vi "Pos ctrl window-Step increment switch.vi"(6 "Mode":enum16{"XY", "Z"}(ring), 9 "State":T1, 10 "Previous State":T1) -> (1 "Wait for acknowledge?":bool, 3 "Increment (um)":sgl)   [LabVIEW 2020]
uses:
  Typedefs/Pos Ctrl States.ctl
  Globals/Pos ctrl window globals.vi
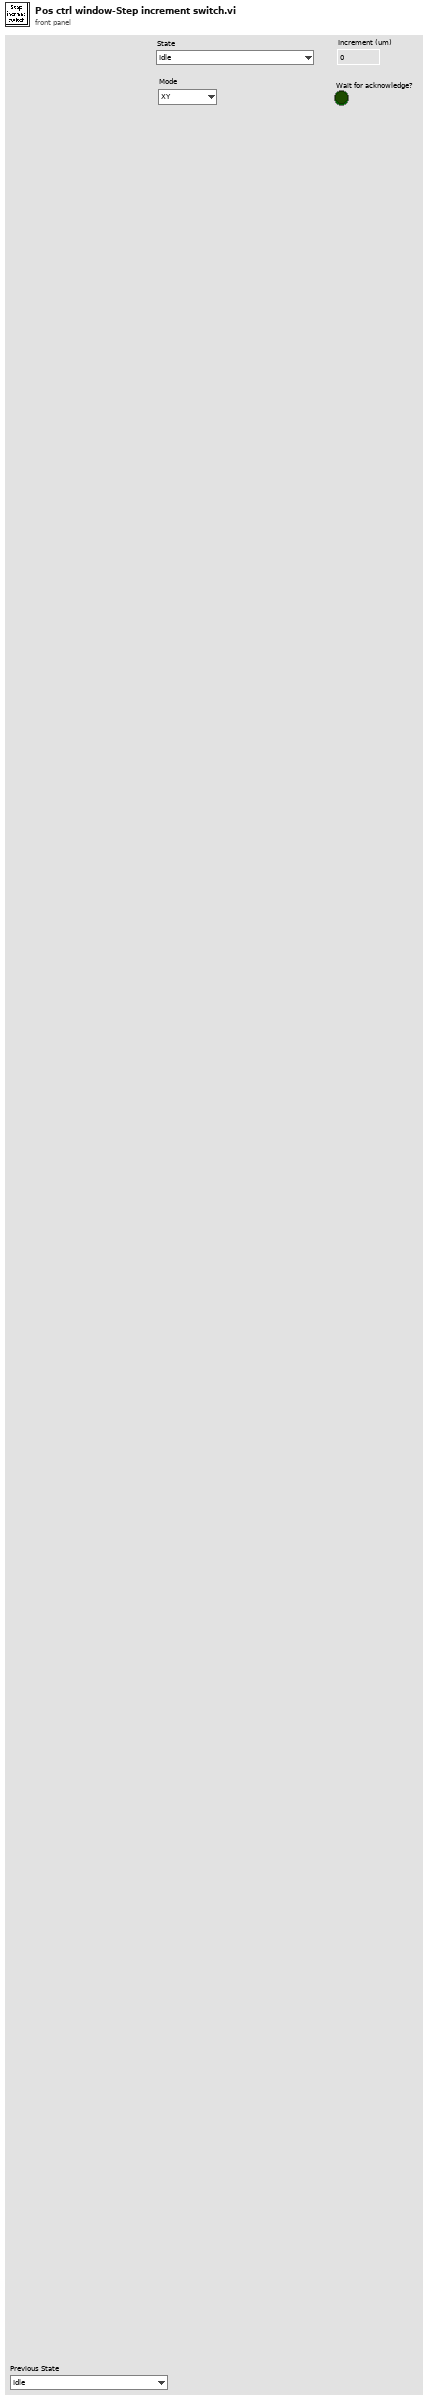
[diagram p1: front panel]
types:
  T1 = typedef "Pos Ctrl States.ctl" = enum16{"Idle", "Count-down", "Request single step (ack.)", "Request single step (no ack.)", "Request continuous movement", "Request movement stop"}
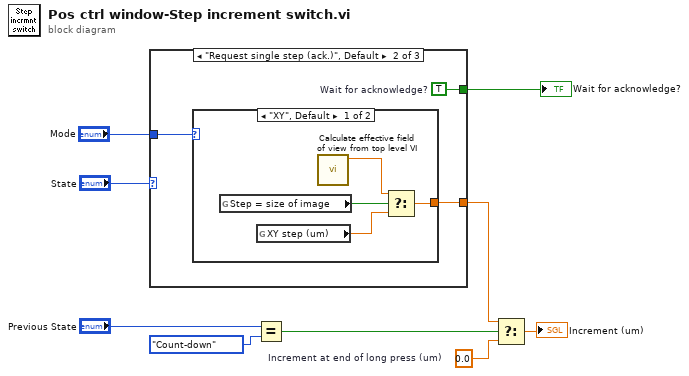
[diagram p0: block diagram]
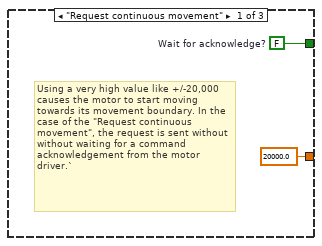
[diagram p2: hidden frame]
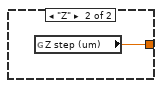
[diagram p3: hidden frame]
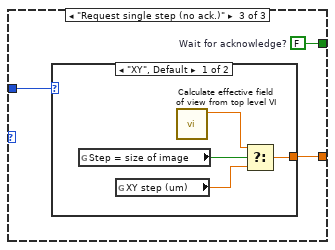
[diagram p4: hidden frame]
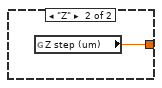
[diagram p5: hidden frame]
diagram:
  w9 = sgl 0.0  # Increment at end of long press (um)
  n1 = case shown="\"Request single step (ack.)\", Default" "State" {
    tunnel: [sgl 20000.0 ("XY step (um)") w14 w22] -> w4
    tunnel: "Mode" -> [_ w13 w21]
    tunnel: [w10 w12 w20] -> w1
    frame "Request continuous movement" {
      w10 = FALSE  # Wait for acknowledge?
      # "Using a very high value like +/-20,000 causes the motor to start moving towards its movement boundary. In the case of the \"Request continuous movement\", the request is sent without without waiting for a command acknowledgement from the motor driver.`"
    }
    frame "Request single step (ack.)", Default {
      w12 = TRUE  # Wait for acknowledge?
      n2 = case shown="\"XY\", Default" w13 {
        tunnel: [w18 w19] -> w14
        frame "XY", Default {
          n3 = global read "Pos ctrl window globals.vi" "Step = size of image"() -> (w16:bool)
          n4 = global read "Pos ctrl window globals.vi" "XY step (um)"() -> (w17:sgl)
          n5 = call "Calculate effective field of view from top level VI.vi"() -> ("Effective FOV (um)"=w15:sgl)  [unwired: 11 in]
          n6 = Select(t=w15, s=w16, f=w17) -> (s? t:f=w18:sgl)
        }
        frame "Z" {
          n7 = global read "Pos ctrl window globals.vi" "Z step (um)"() -> (w19:sgl)
        }
      }
    }
    frame "Request single step (no ack.)" {
      w20 = FALSE  # Wait for acknowledge?
      n8 = case shown="\"XY\", Default" w21 {
        tunnel: [w26 w27] -> w22
        frame "XY", Default {
          n9 = global read "Pos ctrl window globals.vi" "Step = size of image"() -> (w24:bool)
          n10 = global read "Pos ctrl window globals.vi" "XY step (um)"() -> (w25:sgl)
          n11 = call "Calculate effective field of view from top level VI.vi"() -> ("Effective FOV (um)"=w23:sgl)  [unwired: 11 in]
          n12 = Select(t=w23, s=w24, f=w25) -> (s? t:f=w26:sgl)
        }
        frame "Z" {
          n13 = global read "Pos ctrl window globals.vi" "Z step (um)"() -> (w27:sgl)
        }
      }
    }
  }
  "Wait for acknowledge?" <- w1
  n14 = Equal?(x="Previous State", y=Pos_Ctrl_States."Count-down") -> (x = y?=w8:bool)
  n15 = Select(t=w4, s=w8, f=w9) -> (s? t:f=→"Increment (um)":sgl)
